vi "Get Position Names.vi"(11 "Named Positions":T1[](array[typedef])) -> (3 "Array":string[](array[string]))   [LabVIEW 2020, in "Manipulator.lvlib"]
uses:
  Manipulator.lvlib
  Settings/Named Position.ctl
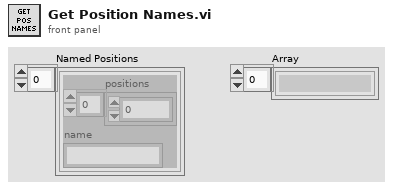
[diagram p1: front panel]
types:
  T1 = typedef "Manipulator.lvlib/Named Position.ctl" = cluster{"positions":dbl[], "name":string}
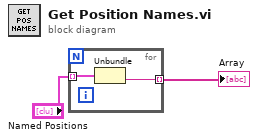
[diagram p0: block diagram]
diagram:
  n1 = for {
    tunnel: "Named Positions" -> [w4] mode=indexing
    tunnel: [w3] -> w2 mode=indexing
    n2 = Unbundle(w4) -> ("name"=w3:string)  [unwired: 1 out]
  }
  "Array" <- w2
